vi "String to dbl System dec point.vi"(11 "n [rpm]":string) -> (3 "Numeric":dbl)   [LabVIEW 2019]
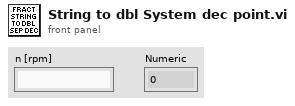
[diagram p1: front panel]
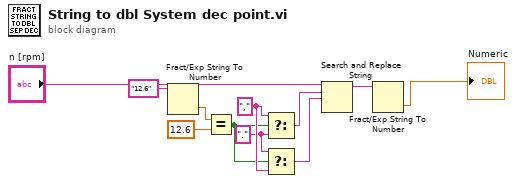
[diagram p0: block diagram]
diagram:
  w8 = "." ("f")
  w9 = ","
  n1 = Fract/Exp String To Number(string="12.6") -> (number=w3:dbl)  [unwired: 3 in, 1 out]
  n2 = Equal?(x=w3, y=12.6) -> (x = y?=w7:bool)
  n3 = Select(t=w9, s=w7, f=w8) -> (s? t:f=w5:string)
  n4 = Select(t=w8, s=w7, f=w9) -> (s? t:f=w6:string)
  n5 = Search and Replace String(input string="n [rpm]", search string=w5, replace string=w6) -> (result string=w10:string)  [unwired: 5 in, 3 out]
  n6 = Fract/Exp String To Number(string=w10) -> (number=→"Numeric":dbl)  [unwired: 3 in, 1 out]
